vi "Stop Stimulator_new.vi"(7 "Stimulator":T1={"Stim Open Data"={"Name"="", "Mode"=enum."LIVE", "Visa Timeout"=0}, "Stim Init Data"={"Frequency"=0.0, "N Factor"=0, "D/T Int"=0.0, "Active Channels"=[], "LF Channels"=[]}, "Stim Update Data"={"Pulse Mode"=[enum."Single"], "Current"=[], "Pulse Dur"=[]}, "Stim Status"={"Open"=FALSE, "On"=FALSE}}) -> (0 "error out":errorcluster, 1 "Log Entry":string, 2 "Response":u8, 3 "Stimulator Out":T1={"Stim Open Data"={"Name"="", "Mode"=enum."LIVE", "Visa Timeout"=0}, "Stim Init Data"={"Frequency"=0.0, "N Factor"=0, "D/T Int"=0.0, "Active Channels"=[], "LF Channels"=[]}, "Stim Update Data"={"Pulse Mode"=[enum."Single"], "Current"=[], "Pulse Dur"=[]}, "Stim Status"={"Open"=FALSE, "On"=FALSE}})   [LabVIEW 2019]
uses:
  Data Type Defs/Stimulator.ctl
  Data Type Defs/Stim Open Data.ctl
  Data Type Defs/Stim Init Data.ctl
  Data Type Defs/Stim Update Data.ctl
  Data Type Defs/Pulse Mode (array).ctl
  Data Type Defs/Stim Status.ctl
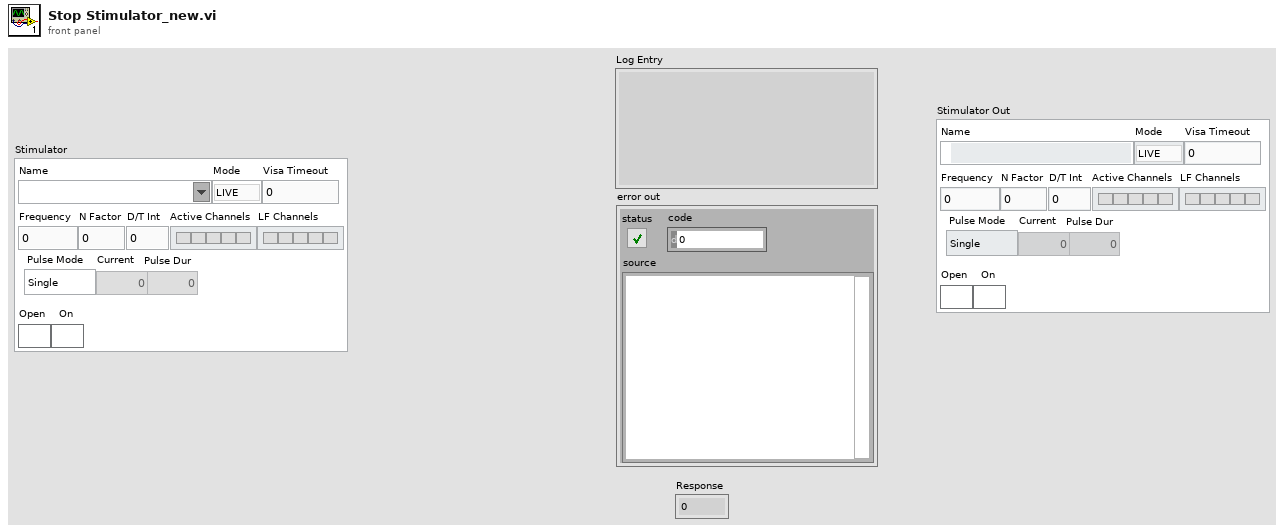
[diagram p1: front panel]
types:
  T1 = typedef "Stimulator.ctl" = cluster{"Stim Open Data":T2, "Stim Init Data":T3, "Stim Update Data":T4, "Stim Status":T6}
  T2 = typedef "Stim Open Data.ctl" = cluster{"Name":refnum<visa-resource-name>, "Mode":enum16{"LIVE", "SIM"}, "Visa Timeout":u32}
  T3 = typedef "Stim Init Data.ctl" = cluster{"Frequency":dbl, "N Factor":u8, "D/T Int":dbl, "Active Channels":bool[], "LF Channels":bool[]}
  T4 = typedef "Stim Update Data.ctl" = cluster{"Pulse Mode":T5, "Current":u32[], "Pulse Dur":u32[]}
  T5 = typedef "Pulse Mode (array).ctl" = enum16{"Single", "Doublet", "Triplet"}[]
  T6 = typedef "Stim Status.ctl" = cluster{"Open":bool, "On":bool}
  T7 = cluster{"Command Name":string, "Command String":string, "Log String":string}
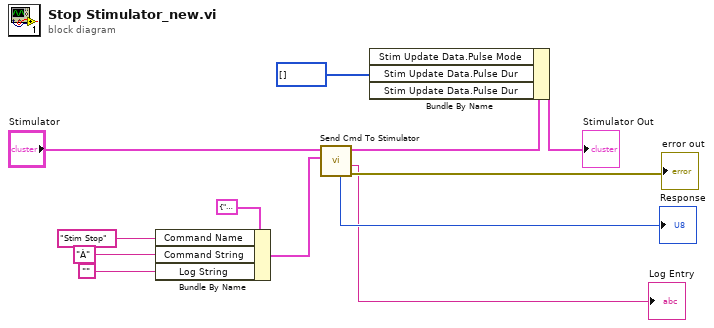
[diagram p0: block diagram]
diagram:
  w7 = i32[] []
  n1 = Bundle By Name(cluster=T7 {"Command Name"="", "Command String"="", "Log String"=""} ("Command"), "Command Name"="Stim Stop", "Command String"="À", "Log String"="") -> (w11:T7)
  n2 = call "Send Cmd To Stimulator.vi"("Stimulator"="Stimulator", "Command"=w11) -> ("Numeric Response"=→"Response":u8, "Stimulator"=w9:T1, "Log Entry"=→"Log Entry":string, "error out"=→"error out":errorcluster)  [unwired: 2 in, 1 out]
  n3 = Bundle By Name(cluster=w9, "Stim Update Data.Pulse Mode"=w7, "Stim Update Data.Pulse Dur"=w7, "Stim Update Data.Pulse Dur"=w7) -> (→"Stimulator Out":T1)
